vi "Julian_project4.vi"() -> ()   [LabVIEW 2020]
doc: "This is a generic calculator for basic arithmetic. Add, subtract, multiply, divide, squareroot, percent, clear, and clear entry functions are implemented."
uses:
  calc_enum.ctl
panel:
  out "Numeric":dbl
  out "?":T1
  out "String":string
  in  "off":bool caption="1"
  in  "clear":bool caption="1"
  in  "clear entry":bool caption="1"
  in  "0":bool caption="1"
  in  "/\n/":bool caption="1"
  in  "*":bool caption="1"
  in  "=":bool caption="1"
  in  "+":bool caption="1"
  in  "%":bool caption="1"
  in  "sqrt":bool caption="1"
  in  "dot":bool caption="1"
  in  "3":bool caption="1"
  in  "6":bool caption="1"
  in  "9":bool caption="1"
  in  "2":bool caption="1"
  in  "1":bool
  in  "5":bool caption="1"
  in  "8":bool caption="1"
  in  "4":bool caption="1"
  in  "7":bool caption="1"
  in  "-":bool caption="1"
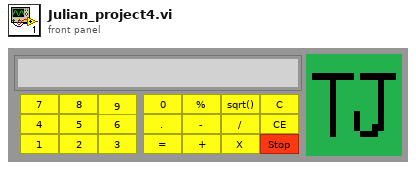
[diagram p1: front panel]
types:
  T1 = typedef "calc_enum.ctl" = enum16{"+", "-", "/", "*", "sqrt", "%"}
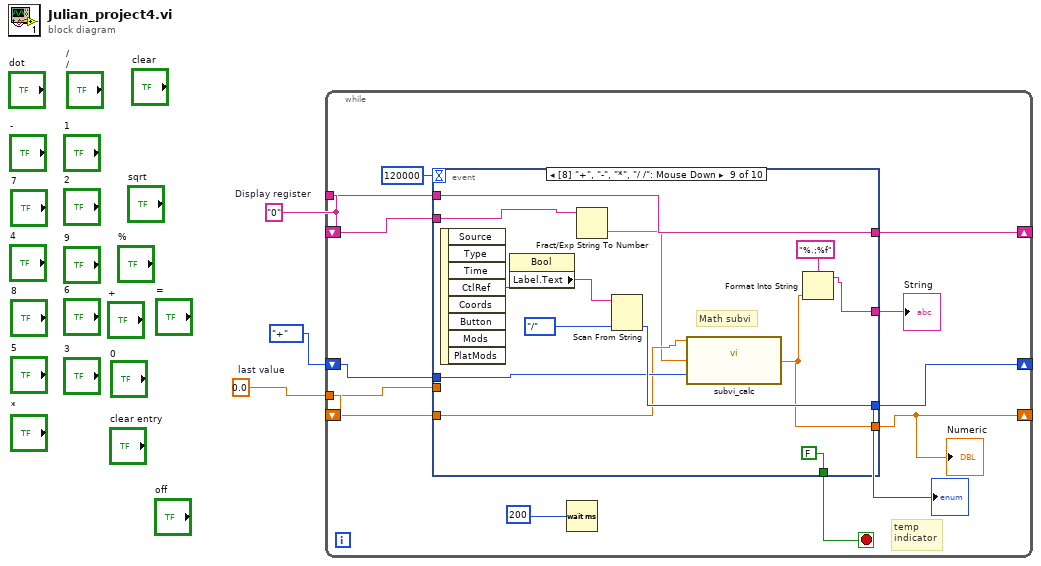
[diagram p0: block diagram]
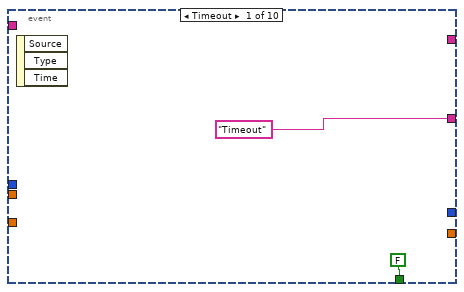
[diagram p2: hidden frame]
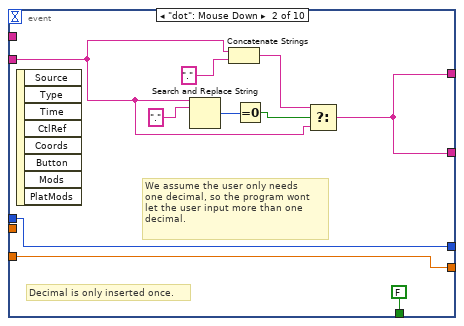
[diagram p3: hidden frame]
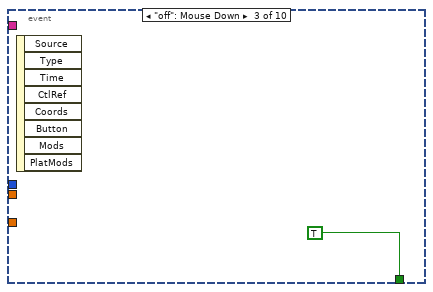
[diagram p4: hidden frame]
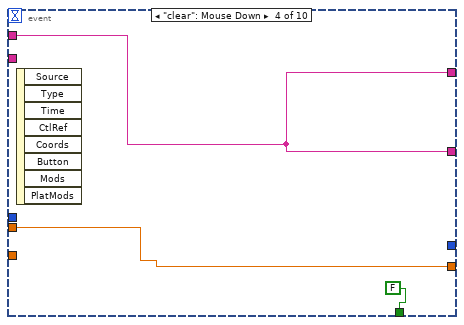
[diagram p5: hidden frame]
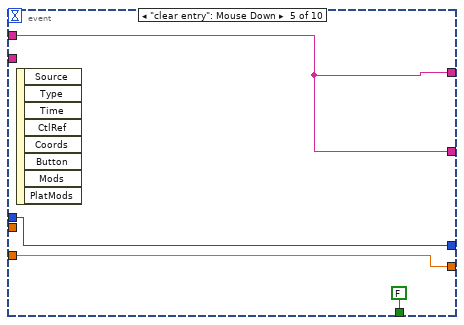
[diagram p6: hidden frame]
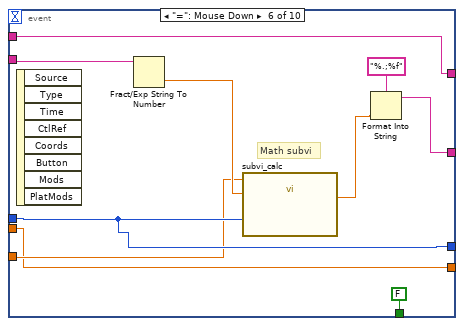
[diagram p7: hidden frame]
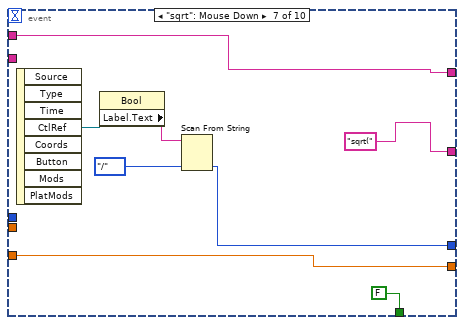
[diagram p8: hidden frame]
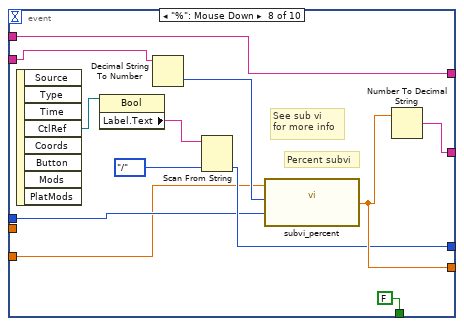
[diagram p9: hidden frame]
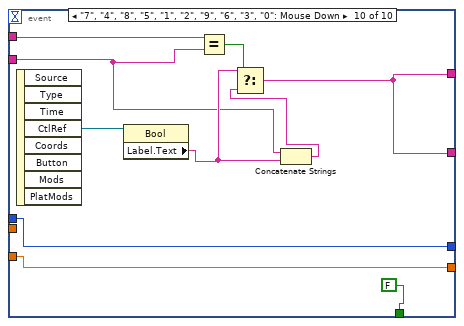
[diagram p10: hidden frame]
diagram:
  w1 = 0.0  # last value
  w3 = "0"  # Display register
  n1 = while {
    shift-right: [w10] -> _
    shift-left: w3 -> [w14]
    tunnel: w3 -> [w12]
    shift-right: [w7] -> _
    shift-left: calc_enum."+" -> [w9]
    shift-right: [w5] -> _
    shift-left: w1 -> [w8]
    tunnel: w1 -> [w4]
    stop <- w6 stop-if-true
    # "temp\nindicator"
    n2 = event shown="[8] \"+\", \"-\", \"*\", \"/ /\": Mouse Down" {
      selector: _ -> [_ _ _ _ _ _ _ _ _ _]
      dyn-events: _ -> [_ _ _ _ _ _ _ _ _ _]
      timeout: 120000 -> [_ _ _ _ _ _ _ _ _ _]
      tunnel: ["Timeout" w21 _ w31 w33 w40 "sqrt(" ("Label.Text") w60 w66 w84] -> w11
      tunnel: w14 -> [_ w22 _ _ _ w44 _ w62 w74 w82]
      tunnel: w12 -> [_ _ _ w31 w33 w37 w51 w61 w72 w83]
      tunnel: [_ w21 _ w31 w33 w37 w51 w61 w72 w84] -> w10
      tunnel: w9 -> [_ w19 _ _ w34 w43 _ w57 w71 w79]
      tunnel: w8 -> [_ w18 _ _ w35 w42 w47 w55 w70 w80]
      tunnel: [_ w18 _ w29 w35 w36 w47 w59 w67 w80] -> w5
      tunnel: [_ w19 _ _ w34 w43 w50 w58 w75 w79] -> w7
      tunnel: [FALSE FALSE TRUE FALSE FALSE FALSE FALSE FALSE FALSE FALSE] -> w6
      tunnel: w4 -> [_ _ _ w29 _ w36 _ _ _ _]
      event Timeout {
        n3 = event-data() -> ()  [unwired: 1 in, 3 out]
      }
      event "dot": Mouse Down {
        # "We assume the user only needs \none decimal, so the program wont\nlet the user input more than one \ndecimal."
        # "Decimal is only inserted once."
        n4 = event-data() -> ()  [unwired: 1 in, 8 out]
        n5 = Search and Replace String(input string=w22, search string=".") -> (number of replacements=w26:i32)  [unwired: 6 in, 3 out]
        n6 = Concatenate Strings(w22, "." ("string")) -> (w24:string)
        n7 = Equal To 0?(x=w26) -> (x = 0?=w25:bool)
        n8 = Select(t=w24, s=w25, f=w22) -> (s? t:f=w21:string)
      }
      event "off": Mouse Down {
        n9 = event-data() -> ()  [unwired: 1 in, 8 out]
      }
      event "clear": Mouse Down {
        n10 = event-data() -> ()  [unwired: 1 in, 8 out]
      }
      event "clear entry": Mouse Down {
        n11 = event-data() -> ()  [unwired: 1 in, 8 out]
      }
      event "=": Mouse Down {
        # "Math subvi"
        n12 = event-data() -> ()  [unwired: 1 in, 8 out]
        n13 = Fract/Exp String To Number(string=w44) -> (number=w45:dbl)  [unwired: 3 in, 1 out]
        n14 = call "subvi_calc.vi"("Function"=w43, "Input in"=w45, "Input 1"=w42) -> ("Answer"=w41:dbl)  [unwired: 8 in]
        n15 = Format Into String(format string="%.;%f", w41) -> (resulting string=w40:string)  [unwired: 2 in, 1 out]
      }
      event "sqrt": Mouse Down {
        n16 = event-data() -> ("CtlRef"=w49:refnum<vi>)  [unwired: 1 in, 7 out]
        n17 = property class="Bool"(reference=w49) -> ("Label.Text"=w53:string)  [unwired: 1 in, 2 out]
        n18 = Scan From String(input string=w53, default 1=calc_enum."/") -> (output 1=w50:T1)  [unwired: 3 in, 3 out]
      }
      event "%": Mouse Down {
        # "See sub vi\nfor more info"
        # "Percent subvi"
        n19 = event-data() -> ("CtlRef"=w56:refnum<vi>)  [unwired: 1 in, 7 out]
        n20 = property class="Bool"(reference=w56) -> ("Label.Text"=w64:string)  [unwired: 1 in, 2 out]
        n21 = Decimal String To Number(string=w62) -> (number=w65:i32)  [unwired: 2 in, 1 out]
        n22 = Scan From String(input string=w64, default 1=calc_enum."/") -> (output 1=w58:T1)  [unwired: 3 in, 3 out]
        n23 = call "subvi_percent.vi"("Function"=w57, "Input in"=w65, "Input 1"=w55) -> ("Answer"=w59:dbl)  [unwired: 8 in]
        n24 = Number To Decimal String(number=w59) -> (decimal integer string=w60:string)  [unwired: 1 in]
      }
      event "+", "-", "*", "/\n/": Mouse Down {
        # "Math subvi"
        n25 = event-data() -> ("CtlRef"=w78:refnum<vi>)  [unwired: 1 in, 7 out]
        n26 = property class="Bool"(reference=w78) -> ("Label.Text"=w77:string)  [unwired: 1 in, 2 out]
        n27 = Fract/Exp String To Number(string=w74) -> (number=w69:dbl)  [unwired: 3 in, 1 out]
        n28 = Scan From String(input string=w77, default 1=calc_enum."/") -> (output 1=w75:T1)  [unwired: 3 in, 3 out]
        n29 = call "subvi_calc.vi"("Function"=w71, "Input in"=w69, "Input 1"=w70) -> ("Answer"=w67:dbl)  [unwired: 8 in]
        n30 = Format Into String(format string="%.;%f", w67) -> (resulting string=w66:string)  [unwired: 2 in, 1 out]
      }
      event "7", "4", "8", "5", "1", "2", "9", "6", "3", "0": Mouse Down {
        n31 = event-data() -> ("CtlRef"=w88:refnum<vi>)  [unwired: 1 in, 7 out]
        n32 = property class="Bool"(reference=w88) -> ("Label.Text"=w86:string)  [unwired: 1 in, 2 out]
        n33 = Equal?(x=w83, y=w82) -> (x = y?=w87:bool)
        n34 = Concatenate Strings(w82, w86) -> (w85:string)
        n35 = Select(t=w86, s=w87, f=w85) -> (s? t:f=w84:string)
      }
    }
    "String" <- w11
    "?" <- w7
    "Numeric" <- w5
    n36 = Wait (ms)(milliseconds to wait=200) -> ()  [unwired: 1 out]
  }
